vi "Acq Fetch Waveform (Complex WDT).vi"(0 "session in":refnum<class "Digitizer Control.lvclass">, 2 "elements to read":u32, 5 "error in (no error)":errorcluster, 7 "timeout (ms)":i32=5000, 8 "channel index":i32, 9 "clear time out error? (F)":bool) -> (13 "timed out?":bool, 14 "session out":refnum<class "Digitizer Control.lvclass">, 15 "waveform (V)":waveform(dbl), 17 "elements remaining":u32, 19 "error out":errorcluster)   [LabVIEW 2021, in "Digitizer Control.lvclass"]
doc: "Fetches the acquired waveform. Use the <B>Acq Configure Channel.vi</B> to configure the channel parameters, the <B>Acq Configure Transfer.vi</B> to configure the waveform transfer, and the <B>Acq Configure Start Trigger.vi</B> to configure the start trigger, then use the <B>Acq Initiate.vi</B> to initiate the acquisition. After the acquisition is initiated, use this VI to fetch the acquired samples. Use the <B>Acq Get Status.vi</B> to check the acquisition status and the <B>Acq Stop.vi</B> to stop an acquisition.\n\nInputs:\n\n<B>session in</B>: The device session.\n\n<B>channel index</B>: The index of the channel to read.\n\n<B>elements to read</B>: The number of elements to read from the host DMA buffer to fetch the acquired samples. For example, in case of a finite acquisition wire the <B>elements to read</B> output of the <B>Acq Initiate.vi</B> to this input. NOTE: This input must be a multiple of the <B>transfer quantum size (elements)</B> value returned by the <B>Acq Configure Transfer.vi</B>.\n\n<B>timeout</B>: The maximum amount of time, in milliseconds, this VI is allowed to wait for the requested number of elements to become available.\n\n<B>clear time out error?</B>: If this input is true, then the <B>error out</B> output does not return the time out error.\n\nOutputs:\n\n<B>session out</B>: The device session passed on the <B>session in</B> input.\n\n<B>waveform</B>: The acquired samples, scaled to Volts.\n\n<B>elements remaining</B>: The number of additional elements remaining in the host DMA buffer that are available for reading.\n\n<B>timed out?</B>: A true on this output indicates that the fetch operation timed out.\n\nNotes:\n\nDo not mix the different Acq Fetch Waveform VIs. Once this VI is called on a channel, use only this VI to fetch the acquired samples on that channel. If you want to use another fetch VI, then it is recommended to reconfigure the transfer first using the <B>Acq Configure Transfer.vi</B>."
uses:
  Digitizer Control.lvclass
  Digitizer Control.lvclass/Digitizer Control.ctl
  <vilib>/Utility/error.llb/Error Cluster From Error Code.vi
  <vilib>/rvi/errors/niLvFpgaAdjustHostInterfaceError.vi
  <vilib>/ErrorRing/Error Ring.xnode
  <vilib>/rvi/interface/nirviMethod/nirviMethod.xnode
  <vilib>/FPGAPlugInAG/Dynamic/niLvFpga_ReadFifo_Dynamic.vi
  <vilib>/rvi/errors/niLvFpgaMergeErrorWithErrorCode.vi
  <vilib>/gmath/NI_Gmath.lvlib
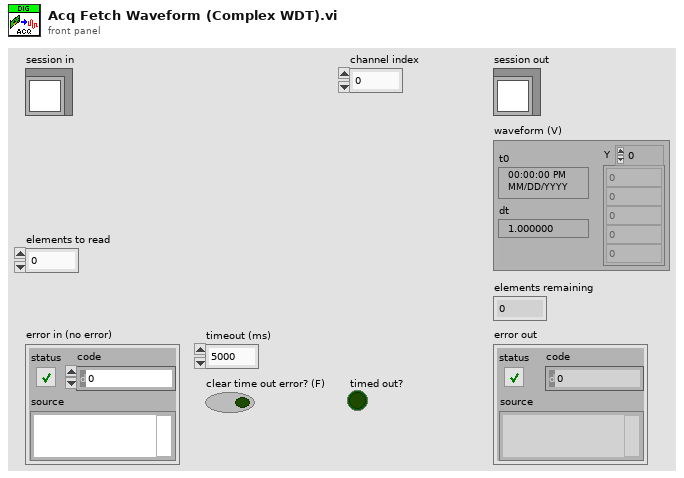
[diagram p1: front panel]
types:
  T1 = typedef "Digitizer Control.lvclass/Acq Session Data.ctl" = cluster{"ADC sampling rate":dbl, "SCTL rate":dbl, "DMA element size (bits)":i32, "sample size (bits)":i32[], "DMA/memory interface width (DMA elements)":i32, "transfer size (bits)":i32[], "stream instance":i32[], "trigger instance":u32, "group delay (s)":dbl, "data delay (s)":dbl, "target delay (s)":dbl, "trigger tracking enabled":bool, "channel configured":bool, "enabled channels":bool[], "transfer configured":bool, "dsp bypass":bool, "fractional decimator input rate":dbl, "fractional decimator output rate":dbl, "sample scale factor":dbl[], "memory size":u64[], "FIFO size":u64}
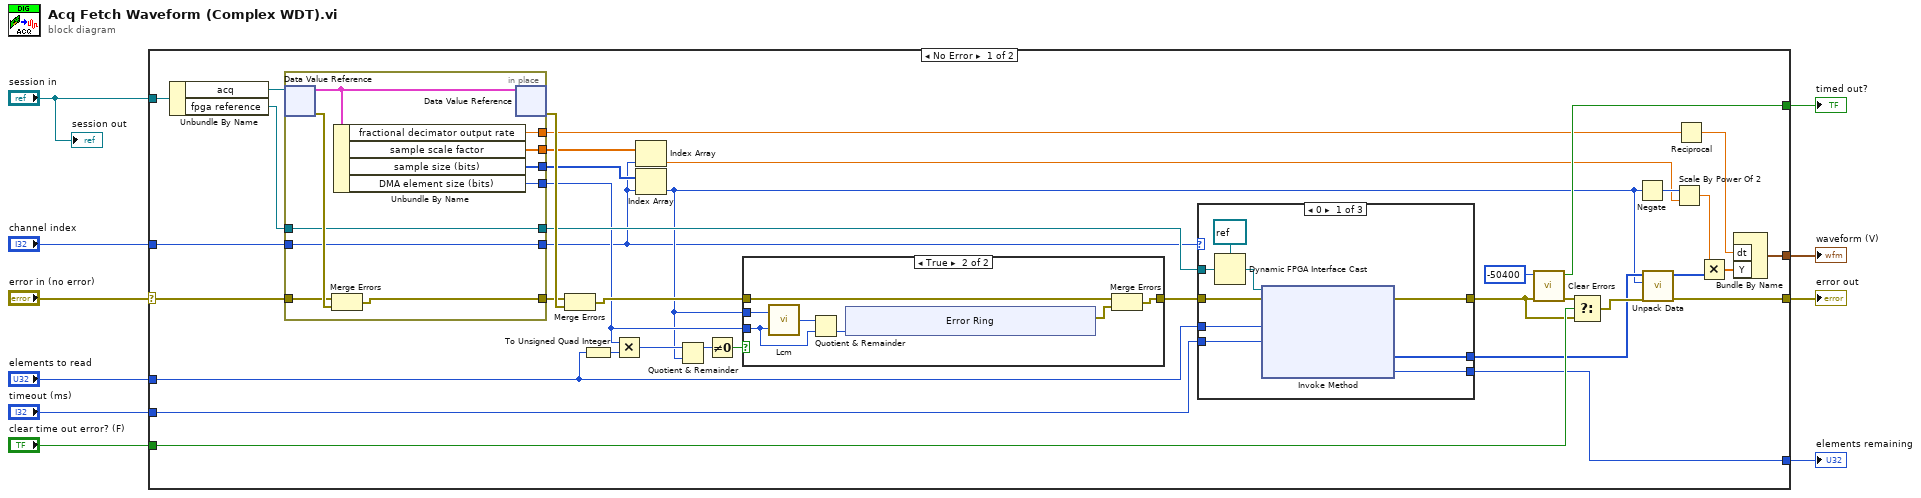
[diagram p0: block diagram]
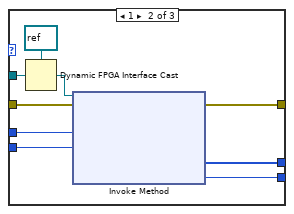
[diagram p2: hidden frame]
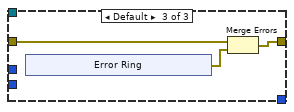
[diagram p3: hidden frame]
diagram:
  n1 = case shown="No Error" "error in (no error)" {
    selector: "error in (no error)" -> [w41 w100]
    tunnel: "elements to read" -> [w26 _]
    tunnel: [w19 w100] -> w4
    tunnel: "timeout (ms)" -> [w44 _]
    tunnel: [w43 _] -> w7
    tunnel: "session in" -> [w36 _]
    tunnel: [w38 _] -> w6
    tunnel: "clear time out error? (F)" -> [w47 _]
    tunnel: [w48 _] -> w2
    tunnel: "channel index" -> [w16 _]
    frame No Error {
      n2 = Unbundle By Name(w36) -> ("acq"=w35:refnum<data-value>, "fpga reference"=w34:refnum<k20>)
      n3 = in-place {
        in-place-border: w41 -> [w98]
        in-place-border: [w96] -> w40
        in-place-border: [w95] -> w13
        in-place-border: [w94] -> w39
        in-place-border: w34 -> [w93]
        in-place-border: [w93] -> w33
        in-place-border: [w92] -> w15
        in-place-border: [w91] -> w27
        in-place-border: w16 -> [w90]
        in-place-border: [w90] -> w11
        n4 = in-place-dvr #1(w35) -> (w97:T1, w99:errorcluster)
        n5 = Merge Errors(w98, w99) -> (w94:errorcluster)
        n6 = Unbundle By Name(w97) -> ("fractional decimator output rate"=w96:dbl, "sample scale factor"=w95:dbl[], "sample size (bits)"=w92:i32[], "DMA element size (bits)"=w91:i32)
        n7 = in-place-dvr #1(w97) -> (w45:errorcluster)  [unwired: 1 out]
      }
      n8 = Merge Errors(w39, w45) -> (w46:errorcluster)
      n9 = To Unsigned Quad Integer(1:w26) -> (0:w25:u64)
      n10 = Multiply(x=w27, y=w25) -> (x*y=w30:u64)
      n11 = Index Array(array=w13, index=w11) -> (element=w12:dbl)
      n12 = Index Array(array=w15, index=w11) -> (element=w14:i32)
      n13 = Quotient & Remainder(x=w30, y=w14) -> (x-y*floor(x/y)=w29:u64)  [unwired: 1 out]
      n14 = Not Equal To 0?(x=w29) -> (x != 0?=w28:bool)
      n15 = case shown="True" w28 {
        tunnel: w46 -> [w75 w82]
        tunnel: [w75 w81] -> w24
        tunnel: w27 -> [_ w77]
        tunnel: w14 -> [_ w79]
        frame False {
        }
        frame True {
          n16 = call <vilib>:"Lcm.vi"("y"=w77, "x"=w79) -> ("lcm(x,y)"=w78:i64)
          n17 = Quotient & Remainder(x=w78, y=w77) -> (floor(x/y)=w76:i64)  [unwired: 1 out]
          n18 = xnode "Error Ring"("parameter 0"=w76) -> ("error out"=w80:errorcluster)
          n19 = Merge Errors(w82, w80) -> (w81:errorcluster)
        }
      }
      n20 = case shown="0" w11 {
        tunnel: w44 -> [w57 w66 _]
        tunnel: [w54 w63 _] -> w38
        tunnel: w33 -> [w53 w62 _]
        tunnel: w26 -> [w52 w61 _]
        tunnel: w24 -> [w51 w60 w68]
        tunnel: [w50 w59 w67] -> w21
        tunnel: [w49 w58 _] -> w18
        frame 0 {
          n21 = Dynamic FPGA Interface Cast(Session In=refnum<k20> refnum ("Type"), Type=w53) -> (Session Out=w56:refnum<k20>)
          n22 = xnode "Invoke Method"("FPGA VI Reference In"=w56, "error in"=w51, "Number of Elements"=w52, "Timeout (ms)"=w57) -> ("error out"=w50:errorcluster, "Data"=w49:i16[], "Elements Remaining"=w54:u32)  [unwired: 1 out]
        }
        frame 1 {
          n23 = Dynamic FPGA Interface Cast(Session In=refnum<k20> refnum ("Type"), Type=w62) -> (Session Out=w65:refnum<k20>)
          n24 = xnode "Invoke Method"("FPGA VI Reference In"=w65, "error in"=w60, "Number of Elements"=w61, "Timeout (ms)"=w66) -> ("error out"=w59:errorcluster, "Data"=w58:i16[], "Elements Remaining"=w63:u32)  [unwired: 1 out]
        }
        frame Default {
          n25 = xnode "Error Ring"() -> ("error out"=w69:errorcluster)
          n26 = Merge Errors(w68, w69) -> (w67:errorcluster)
        }
      }
      n27 = call <vilib>:"Clear Errors.vi"("error in (no error)"=w21, "specific error code to clear (0: all)"=-50400) -> ("error out"=w22:errorcluster, "specific error cleared?"=w48:bool)  [unwired: 4 in]
      n28 = Select(t=w22, s=w47, f=w21) -> (s? t:f=w20:errorcluster)
      n29 = Negate(x=w14) -> (-x=w32:i32)
      n30 = call "Unpack Data.vi"("error in (no error)"=w20, "packed data size (bits)"=w14, "packed data in"=w18) -> ("error out"=w19:errorcluster, "unpacked data out"=w17:i16[])  [unwired: 7 in]
      n31 = Scale By Power Of 2(n=w32, x=w12) -> (x*2^n=w31:dbl)
      n32 = Reciprocal(x=w40) -> (1/x=w37:dbl)
      n33 = Multiply(x=w31, y=w17) -> (x*y=w42:dbl[])
      n34 = Bundle By Name("dt"=w37, "Y"=w42) -> (w43:waveform(dbl))  [unwired: 1 in]
    }
    frame Error {
    }
  }
  "waveform (V)" <- w7
  "elements remaining" <- w6
  "error out" <- w4
  "timed out?" <- w2
  "session out" <- "session in"
